vi "variable_settings_to_string.vi"(8 "error in":errorcluster, 11 "Variable Settings":T1={"Measurements per Iteration"=1, "Local Data Path"=path "C:/Users/Saffmanlab/Documents/Cesium/data", "Experiment description suffix for filename (no spaces please)"="", "Network Data Path"=path "Z:/", "Copy data to network"=TRUE, "Measurement Timeout (ms)"=0, "Variables"=[], "Parameters"=[], "Run Test Mode"=FALSE} {"Variables"."# steps" min=1 step=1; "Measurements per Iteration" min=1 step=1}) -> (0 "error out":errorcluster, 3 "varible settings string":string)   [LabVIEW 2013, in "ExperimentVariables.lvclass"]
uses:
  ExperimentVariables/ExperimentVariables.lvclass
  ExperimentVariables/Variable_Settings.ctl
panel:
  # "Parameters will be evaluated once at the beginning of the experiment from top to bottom, \nso any parameter may depend on all those above it.\nVariables will be evaluated each iteration.\nParameters and Variables may be used in various other experiment settings, as noted.\nSee LabView Help -> Formula Node and Expression Node Functions for a list of available functions."
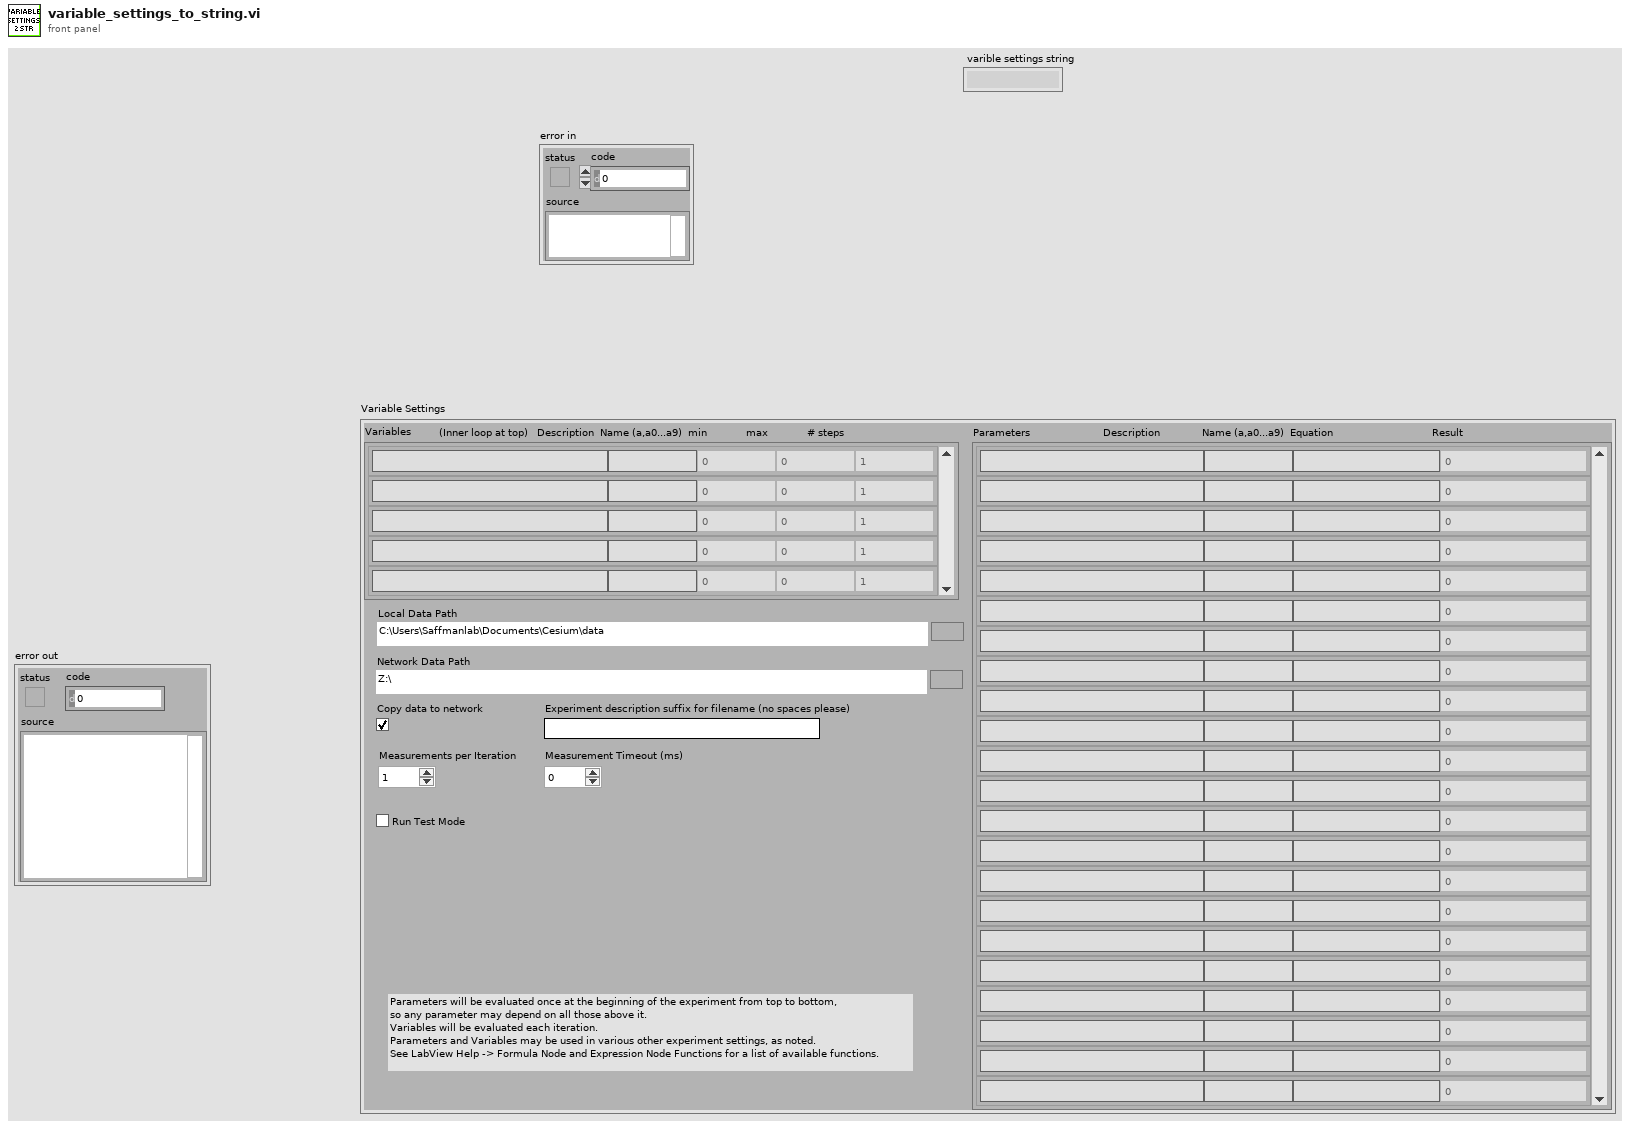
[diagram p1: front panel]
types:
  T1 = typedef "ExperimentVariables.lvclass/Variable_Settings.ctl" = cluster{"Measurements per Iteration":i32, "Local Data Path":path, "Experiment description suffix for filename (no spaces please)":string, "Network Data Path":path, "Copy data to network":bool, "Measurement Timeout (ms)":u32, "Variables":cluster{"Description":string, "Name (a,a0...a9)":string, "min":dbl, "max":dbl, "# steps":u32}[], "Parameters":cluster{"Description":string, "Name (a,a0...a9)":string, "Equation":string, "Result":dbl}[], "Run Test Mode":bool}
  T2 = cluster{"Description":string, "Name (a,a0...a9)":string, "Equation":string, "Result":dbl}[]
  T3 = cluster{"Description":string, "Name (a,a0...a9)":string, "min":dbl, "max":dbl, "# steps":u32}[]
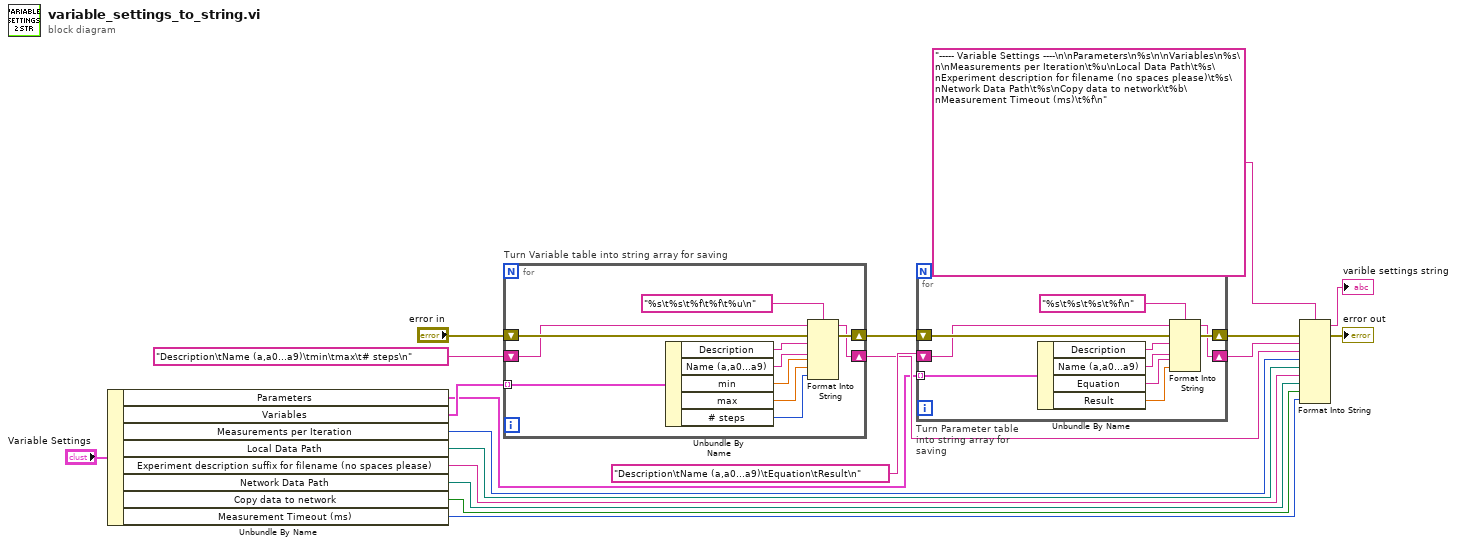
[diagram p0: block diagram]
diagram:
  n1 = Unbundle By Name("Variable Settings") -> ("Parameters"=w1:T2, "Variables"=w2:T3, "Measurements per Iteration"=w5:i32, "Local Data Path"=w18:path, "Experiment description suffix for filename (no spaces please)"=w17:string, "Network Data Path"=w16:path, "Copy data to network"=w15:bool, "Measurement Timeout (ms)"=w14:u32)
  n2 = for "Turn Variable table into string array for saving" {
    tunnel: w2 -> [w23] mode=indexing
    shift-right: [w26] -> w19
    shift-left: "error in" -> [w27]
    shift-right: [w25] -> w3
    shift-left: "Description\tName (a,a0...a9)\tmin\tmax\t# steps\n" ("new element/subarray") -> [w20]
    n3 = Unbundle By Name(w23) -> ("Description"=w21:string, "Name (a,a0...a9)"=w22:string, "min"=w29:dbl, "max"=w28:dbl, "# steps"=w24:u32)
    n4 = Format Into String(format string="%s\t%s\t%f\t%f\t%u\n", initial string=w20, error in=w27, w21, w22, w29, w28, w24) -> (resulting string=w25:string, error out=w26:errorcluster)
  }
  n5 = for "Turn Parameter table into string array for saving" {
    tunnel: w1 -> [w40] mode=indexing
    shift-right: [w35] -> w10
    shift-left: w19 -> [w36]
    shift-right: [w34] -> w4
    shift-left: "Description\tName (a,a0...a9)\tEquation\tResult\n" ("new element/subarray") -> [w31]
    n6 = Unbundle By Name(w40) -> ("Description"=w32:string, "Name (a,a0...a9)"=w33:string, "Equation"=w38:string, "Result"=w37:dbl)
    n7 = Format Into String(format string="%s\t%s\t%s\t%f\n", initial string=w31, error in=w36, w32, w33, w38, w37) -> (resulting string=w34:string, error out=w35:errorcluster)
  }
  n8 = Format Into String(format string="----- Variable Settings ----\n\nParameters\n%s\n\nVariables\n%s\n\nMeasurements per Iteration\t%u\nLocal Data Path\t%s\nExperiment description for filename (no spaces please)\t%s\nNetwork Data Path\t%s\nCopy data to network\t%b\nMeasurement Timeout (ms)\t%f\n", error in=w10, w4, w3, w5, w18, w17, w16, w15, w14) -> (resulting string=→"varible settings string":string, error out=→"error out":errorcluster)  [unwired: 1 in]
